vi "Set Carriers.vi"(8 "error in (no error)":errorcluster, 11 "MCCW ACLR in":refnum<class "MCCW ACLR.lvclass">) -> (0 "error out":errorcluster, 1 "Parameter":cluster{"Name":string, "Value":string}, 2 "Last Carrier?":bool, 3 "MCCW ACLR out":refnum<class "MCCW ACLR.lvclass">)   [LabVIEW 2020, in "MCCW ACLR.lvclass"]
uses:
  MCCW ACLR.lvclass
  MCCW ACLR.lvclass/MCCW ACLR.ctl
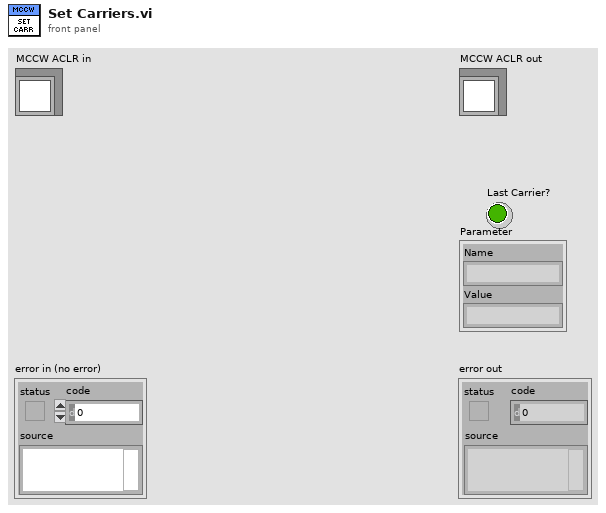
[diagram p1: front panel]
types:
  T1 = cluster{"List":dbl[], "Index":i32, "Last":bool, "BW [MHz]":dbl}
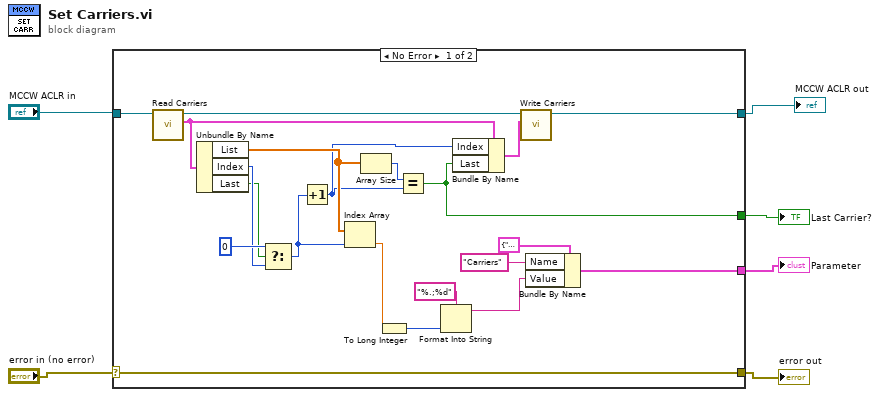
[diagram p0: block diagram]
diagram:
  n1 = case shown="No Error" "error in (no error)" {
    selector: "error in (no error)" -> [w9 w29]
    tunnel: [w9 w29] -> w5
    tunnel: [w10 w28] -> w3
    tunnel: "MCCW ACLR in" -> [w8 w28]
    tunnel: [w17 _] -> w2
    tunnel: [w11 _] -> w1
    frame No Error {
      n2 = call "Read Carriers.vi"("MCCW ACLR in"=w8) -> ("Carriers"=w26:T1, "MCCW ACLR out"=w27:refnum<class "MCCW ACLR.lvclass">)  [unwired: 9 in]
      n3 = Unbundle By Name(w26) -> ("List"=w21:dbl[], "Index"=w24:i32, "Last"=w22:bool)
      n4 = Select(t=0, s=w22, f=w24) -> (s? t:f=w19:i32)
      n5 = Increment(x=w19) -> (x+1=w18:i32)
      n6 = Index Array(array=w21, index=w19) -> (element=w12:dbl)
      n7 = Array Size(array=w21) -> (size(s)=w20:i32)
      n8 = To Long Integer(number=w12) -> (32bit integer=w7:i32)
      n9 = Equal?(x=w20, y=w18) -> (x = y?=w17:bool)
      n10 = Format Into String(format string="%.;%d", w7) -> (resulting string=w13:string)  [unwired: 2 in, 1 out]
      n11 = Bundle By Name(cluster=w26, "Index"=w18, "Last"=w17) -> (w23:T1)
      n12 = call "Write Carriers.vi"("Carriers"=w23, "MCCW ACLR in"=w27) -> ("MCCW ACLR out"=w10:refnum<class "MCCW ACLR.lvclass">)  [unwired: 9 in]
      n13 = Bundle By Name(cluster=cluster{"Name":string, "Value":string} {"Name"="", "Value"=""} ("Change"), "Name"="Carriers", "Value"=w13) -> (w11:cluster{"Name":string, "Value":string})
    }
    frame Error {
    }
  }
  "error out" <- w5
  "MCCW ACLR out" <- w3
  "Last Carrier?" <- w2
  "Parameter" <- w1
